vi "Read Numeric Assertion Type.vi"(8 "error in (no error)":errorcluster, 11 "Numeric Assertion in":refnum<class "Numeric Assertion.lvclass">) -> (0 "error out":errorcluster, 2 "Numeric Assertion Type":T1, 3 "Numeric Assertion out":refnum<class "Numeric Assertion.lvclass">)   [LabVIEW 2020, in "MacroAssert.lvlib" / "Numeric Assertion.lvclass"]
uses:
  Numeric Assertion.lvclass
  Numeric Assertion Type.ctl
  Numeric Assertion.lvclass/Numeric Assertion.ctl
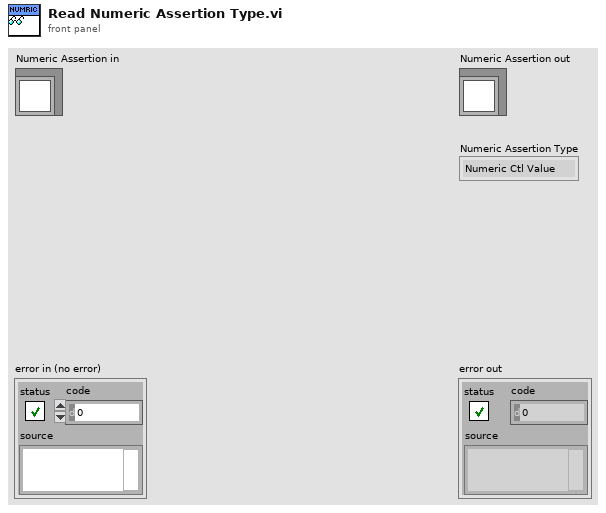
[diagram p1: front panel]
types:
  T1 = typedef "MacroAssert.lvlib/Numeric Assertion.lvclass/Numeric Assertion Type.ctl" = enum16{"Numeric Ctl Value", "Ctl Width Property", "Ctl Height Property", "VI Width", "VI Height", "Window Width", "Window Height"}
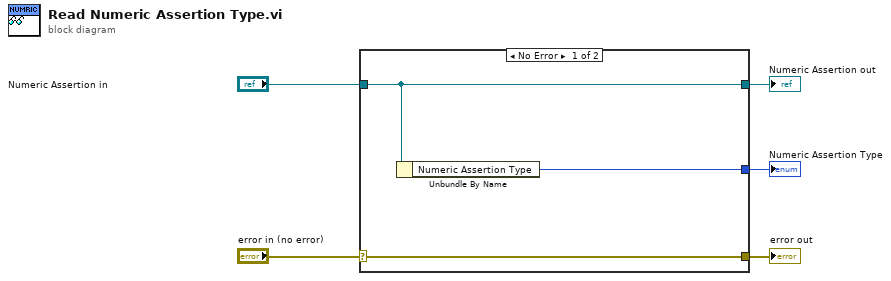
[diagram p0: block diagram]
diagram:
  n1 = case shown="No Error" "error in (no error)" {
    selector: "error in (no error)" -> [w8 w9]
    tunnel: [w8 w9] -> w4
    tunnel: [w7 w10] -> w2
    tunnel: "Numeric Assertion in" -> [w7 w10]
    tunnel: [w6 _] -> w1
    frame No Error {
      n2 = Unbundle By Name(w7) -> ("Numeric Assertion Type"=w6:T1)
    }
    frame Error {
    }
  }
  "error out" <- w4
  "Numeric Assertion out" <- w2
  "Numeric Assertion Type" <- w1
